vi "Self-Test.vi"(0 "VISA resource name":refnum<visa-resource-name>, 11 "error in (no error)":errorcluster) -> (4 "VISA resource name out":refnum<visa-resource-name>, 8 "Self-Test Error":u32, 10 "Self-Test Response":string, 15 "error out":errorcluster)   [LabVIEW 2012, in "Lake Shore Cryotronics 218.lvlib"]
doc: "This VI causes the instrument to perform a self-test and returns the results. A numeric indicator indicates if the instrument passed all self-tests, and a string indicator contains the instrument's reponse. If a self test is not supported, the VI returns a warning code."
uses:
  <instrlib>/Lake Shore Cryotronics 218/Lake Shore Cryotronics 218.lvlib
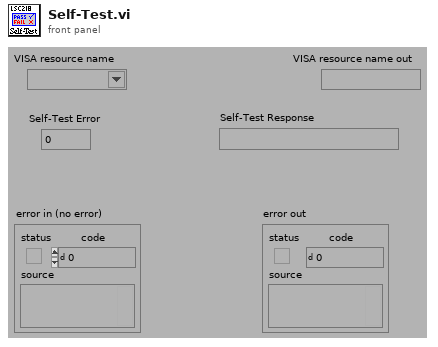
[diagram p1: front panel]
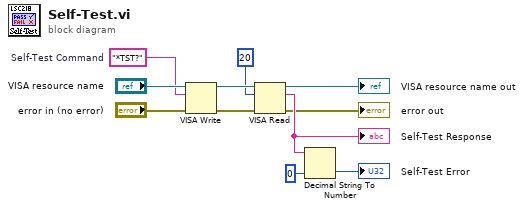
[diagram p0: block diagram]
diagram:
  w2 = "*TST?"  # Self-Test Command
  n1 = VISA Write(VISA resource name="VISA resource name", write buffer=w2, error in (no error)="error in (no error)") -> (VISA resource name out=w5:refnum<visa-resource-name>, error out=w3:errorcluster)  [unwired: 1 out]
  n2 = VISA Read(VISA resource name=w5, byte count=u32 20, error in (no error)=w3) -> (VISA resource name out=→"VISA resource name out":refnum<visa-resource-name>, read buffer=w11:string, error out=→"error out":errorcluster)  [unwired: 1 out]
  "Self-Test Response" <- w11
  n3 = Decimal String To Number(string=w11, default (0L)=u32 0 ("Default (0L)")) -> (number=→"Self-Test Error":u32)  [unwired: 1 in, 1 out]
